vi "Keithley 6514 Voltage Config.vi"(0 "Resource In":refnum<visa-resource-name>, 1 "Check For SCPI Errors? (T)":bool=TRUE, 2 "Driven Guard (Off:F)":bool, 3 "External Feedback (Disabled:F)":bool, 5 "NPLC value (1.00)":dbl=1.0 min=0.01 max=10.0 step=0.01 format="%.2f", 7 "range (autorange:0)":u16(ring) items=["autorange", "set min range", "set max range", "set range value"], 9 "range value (V) (21)":sgl=21.0 min=0 max=210 step=0.1 format="%.2f", 11 "error in (no error)":T1, 12 "Autorange Upper Limit (V) (210)":sgl=210.0 min=0 max=210 step=0.1 format="%^.2e", 13 "Autorange Lower Limit (V) (2.1)":sgl=2.1 min=0 max=210 step=0.1 format="%^.2e") -> (4 "Resource Out (dupl)":refnum<visa-resource-name>, 15 "error out":T1)   [LabVIEW 2014, in "KE6514Driver.lvlib"]
doc: "This VI is used to configure the settings for voltage measurements.\n\nNPLC:\n0.01 to 10\n\nDriven Guard:\nTRUE = on\nFALSE = Off\n\nExternal Feedback:\nTRUE = Enabled\nFALSE = Disabled\n\nRange:\n0 = Autoranging\n1 = Set minimum range\n2 = Set maximum range\n3 = Set range by value\n\nRange value:\n0 to 210\n\nAutorange Upper Limit:\n0 to 210 (210 default)\n\nAutorange Lower Limit:\n0 to 2.1 (2.1 default)"
uses:
  KE6514Driver.lvlib
panel:
  # "on\noff"
  # "Enabled\nDisabled"
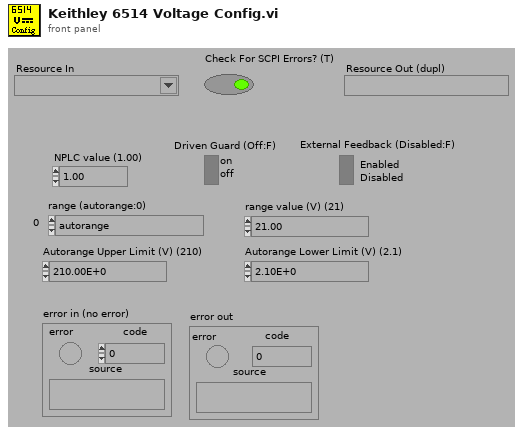
[diagram p1: front panel]
types:
  T1 = cluster{"error":bool, "code":i32, "source":string}
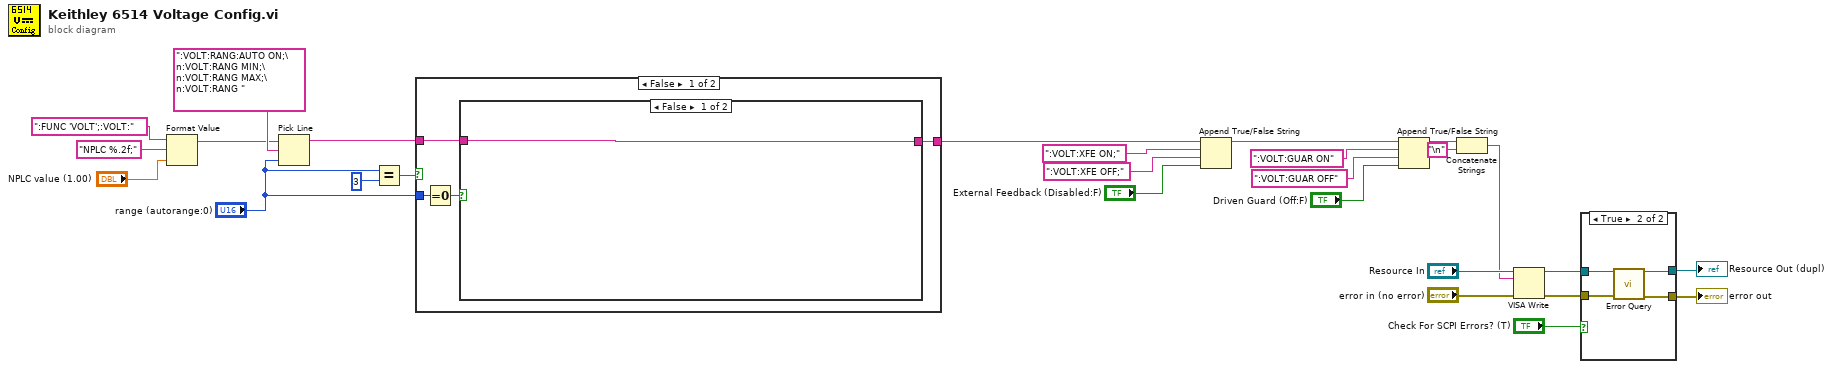
[diagram p0: block diagram]
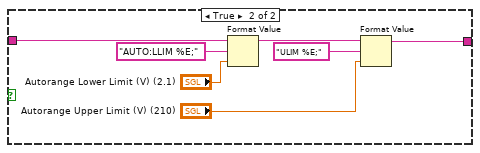
[diagram p3: hidden frame]
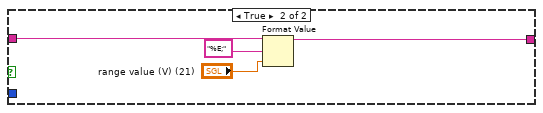
[diagram p4: hidden frame]
diagram:
  n1 = Format Value(string ("")=":FUNC 'VOLT';:VOLT:", format string="NPLC %.2f;", value (0)="NPLC value (1.00)") -> (output string=w17:string)
  n2 = Pick Line(string ("")=w17, multi-line string=":VOLT:RANG:AUTO ON;\n:VOLT:RANG MIN;\n:VOLT:RANG MAX;\n:VOLT:RANG ", line index="range (autorange:0)") -> (output string=w27:string)
  n3 = Equal?(x="range (autorange:0)", y=u16 3) -> (x = y?=w26:bool)
  n4 = case shown="False" w26 {
    tunnel: w27 -> [w28 w42]
    tunnel: [w31 w41] -> w16
    tunnel: "range (autorange:0)" -> [w30 _]
    frame False {
      n5 = Equal To 0?(x=w30) -> (x = 0?=w29:bool)
      n6 = case shown="False" w29 {
        tunnel: [w32 w38] -> w31
        tunnel: w28 -> [w32 w35]
        frame False {
        }
        frame True {
          n7 = Format Value(string ("")=w35, format string="AUTO:LLIM %E;", value (0)="Autorange Lower Limit (V) (2.1)") -> (output string=w39:string)
          n8 = Format Value(string ("")=w39, format string="ULIM %E;", value (0)="Autorange Upper Limit (V) (210)") -> (output string=w38:string)
        }
      }
    }
    frame True {
      n9 = Format Value(string ("")=w42, format string="%E;", value (0)="range value (V) (21)") -> (output string=w41:string)
    }
  }
  n10 = Append True/False String(1:"External Feedback (Disabled:F)", 2:":VOLT:XFE OFF;", 3:":VOLT:XFE ON;", 4:w16) -> (0:w14:string)
  n11 = Append True/False String(1:"Driven Guard (Off:F)", 2:":VOLT:GUAR OFF", 3:":VOLT:GUAR ON", 4:w14) -> (0:w10:string)
  n12 = Concatenate Strings(w10, "\n") -> (w8:string)
  n13 = VISA Write(VISA resource name="Resource In", write buffer=w8, error in (no error)="error in (no error)") -> (VISA resource name out=w4:refnum<visa-resource-name>, error out=w3:errorcluster)  [unwired: 1 out]
  n14 = case shown="True" "Check For SCPI Errors? (T)" {
    tunnel: w4 -> [w45 w49]
    tunnel: w3 -> [w44 w48]
    tunnel: [w45 w47] -> w2
    tunnel: [w44 w46] -> w1
    frame False {
    }
    frame True {
      n15 = call "Error Query.vi"("VISA Resource In"=w49, "error in (no error)"=w48) -> ("VISA Resource Out (dupl)"=w47:refnum<visa-resource-name>, "error out"=w46:errorcluster)  [unwired: 10 in, 2 out]
    }
  }
  "error out" <- w1
  "Resource Out (dupl)" <- w2
